vi "Request CORE.vi"(4 "Timeout":i32, 5 "Answer UE":refnum<user-event>, 6 "Response":bool, 7 "Write":refnum<queue>, 8 "Error In":errorcluster, 9 "Data":string, 10 "Function ID":u8, 11 "Stack ID":u8) -> (0 "Error Out":errorcluster, 1 "timed out":bool, 2 "Sucessful":bool, 3 "Answer":T1)   [LabVIEW 2011, in "Tinkerforge.lvlib" / "IP Connection.lvclass"]
doc: "This VI encapsulates the Request handling for the device class."
uses:
  IP Connection.lvclass
  Type Definitions/Message.ctl
  Type Definitions/Answer.ctl
  Type Definitions/Request Type.ctl
  Type Definitions/Errors.ctl
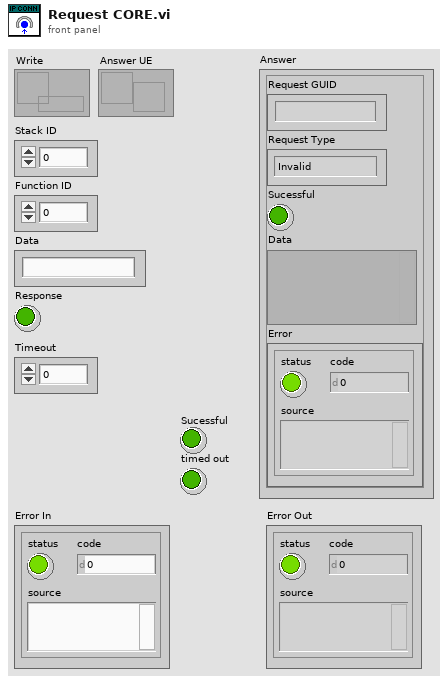
[diagram p1: front panel]
types:
  T1 = typedef "Tinkerforge.lvlib/IP Connection.lvclass/Answer.ctl" = cluster{"Request GUID":string, "Request Type":T2, "Sucessful":bool, "Data":variant, "Error":errorcluster}
  T2 = typedef "Tinkerforge.lvlib/IP Connection.lvclass/Request Type.ctl" = enum8{"Invalid", "Write"}
  T3 = typedef "Tinkerforge.lvlib/IP Connection.lvclass/Errors.ctl" = enum16{"Timeout", "Device type incorrect", "Device already added", "Device not existing"}
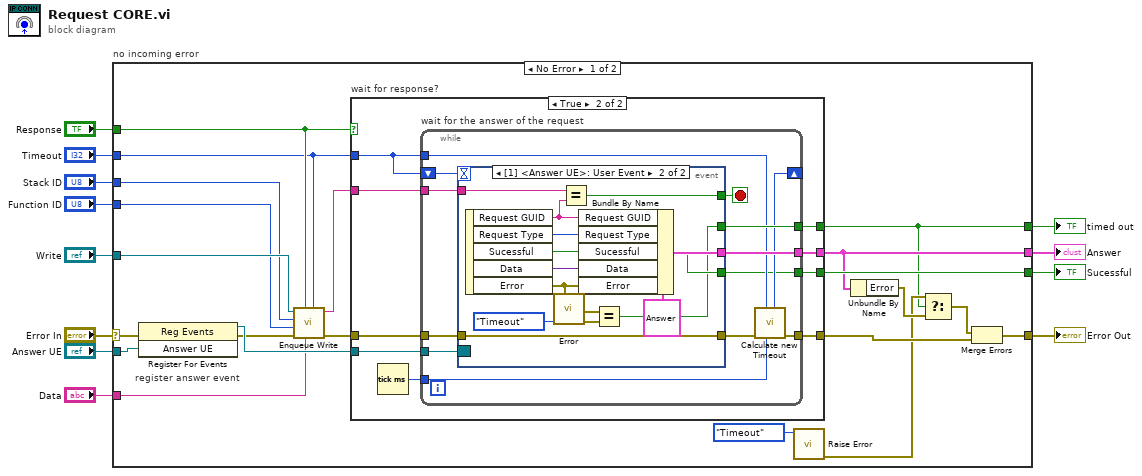
[diagram p0: block diagram]
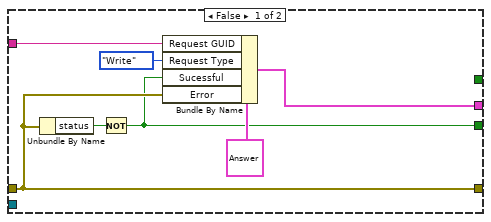
[diagram p2: hidden frame]
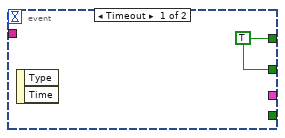
[diagram p3: hidden frame]
diagram:
  n1 = case "no incoming error" shown="No Error" "Error In" {
    selector: "Error In" -> [w29 w77]
    tunnel: [w19 w77] -> w11
    tunnel: "Write" -> [w28 _]
    tunnel: "Answer UE" -> [w33 _]
    tunnel: [w21 _] -> w8
    tunnel: [w14 _] -> w7
    tunnel: "Response" -> [w23 _]
    tunnel: "Stack ID" -> [w26 _]
    tunnel: "Data" -> [w25 _]
    tunnel: "Function ID" -> [w24 _]
    tunnel: "Timeout" -> [w18 _]
    tunnel: [w22 _] -> w1
    frame No Error {
      # "register answer event"
      n2 = register-events(error in=w29, w33) -> (reference out=w32:refnum<event-registration>, error out=w31:errorcluster)  [unwired: 1 in]
      n3 = call "Enqueue Write.vi"("Timeout"=w18, "Data"=w25, "Response"=w23, "error in (no error)"=w31, "Function ID"=w24, "Stack ID"=w26, "Write"=w28) -> ("error out"=w30:errorcluster, "GUID"=w27:string)  [unwired: 3 in]
      n4 = case "wait for response?" shown="True" w23 {
        tunnel: w32 -> [_ w49]
        tunnel: [w36 w48] -> w21
        tunnel: [_ w47] -> w14
        tunnel: [w38 w45] -> w20
        tunnel: w30 -> [w38 w44]
        tunnel: w27 -> [w40 w43]
        tunnel: w18 -> [_ w42]
        tunnel: [w34 w41] -> w22
        frame False {
          n5 = Unbundle By Name(w38) -> ("status"=w35:bool)
          n6 = Not(x=w35) -> (.not. x?=w34:bool)
          n7 = Bundle By Name(cluster=T1 {"Request GUID"="", "Request Type"=enum."Invalid", "Sucessful"=FALSE, "Data"=variant, "Error"={"status"=FALSE, "code"=0, "source"=""}} ("Answer"), "Request GUID"=w40, "Request Type"=Request_Type."Write", "Sucessful"=w34, "Error"=w38) -> (w36:T1)
        }
        frame True {
          n8 = Tick Count (ms)() -> (millisecond timer value=w46:u32)
          n9 = while "wait for the answer of the request" {
            tunnel: w44 -> [w60]
            tunnel: w49 -> [w62]
            shift-right: [w51] -> _
            shift-left: w42 -> [w61]
            tunnel: w43 -> [w59]
            tunnel: [w57] -> w48
            tunnel: [w56] -> w47
            tunnel: w46 -> [w53]
            tunnel: [w54] -> w45
            tunnel: w42 -> [w52]
            tunnel: [w50] -> w41
            stop <- w58 stop-if-true
            n10 = event shown="[1] <Answer UE>: User Event" {
              selector: w62 -> [_ _]
              dyn-events: _ -> [_ _]
              timeout: w61 -> [_ _]
              tunnel: w60 -> [_ w69]
              tunnel: w59 -> [_ w76]
              tunnel: [w63 w75] -> w58
              tunnel: [_ w70] -> w57
              tunnel: [w63 w64] -> w56
              tunnel: [_ w69] -> w55
              tunnel: [_ w68] -> w50
              event Timeout {
                w63 = TRUE
                n11 = event-data() -> ()  [unwired: 1 in, 2 out]
              }
              event User Event {
                n12 = event-data() -> ("Request GUID"=w73:string, "Request Type"=w72:T2, "Sucessful"=w68:bool, "Data"=w71:variant, "Error"=w67:errorcluster)  [unwired: 1 in]
                n13 = call "Error.vi"("Error"=Errors."Timeout") -> ("error cluster"=w65:errorcluster)  [unwired: 10 in]
                n14 = Equal?(x=w76, y=w73) -> (x = y?=w75:bool)
                n15 = Bundle By Name(cluster=T1 {"Request GUID"="", "Request Type"=enum."Invalid", "Sucessful"=FALSE, "Data"=variant, "Error"={"status"=FALSE, "code"=0, "source"=""}} ("Answer"), "Request GUID"=w73, "Request Type"=w72, "Sucessful"=w68, "Data"=w71, "Error"=w67) -> (w70:T1)
                n16 = Equal?(x=w67, y=w65) -> (x = y?=w64:bool)
              }
            }
            n17 = call "Calculate new Timeout.vi"("Start Time"=w53, "Total Timeout"=w52, "Error In"=w55) -> ("Error Out"=w54:errorcluster, "remaining Timeout"=w51:i32)  [unwired: 7 in]
          }
        }
      }
      n18 = call "Raise Error.vi"("Error"=Errors."Timeout") -> ("Error Out"=w15:errorcluster)  [unwired: 10 in]
      n19 = Unbundle By Name(w21) -> ("Error"=w17:errorcluster)
      n20 = Select(t=w15, s=w14, f=w17) -> (s? t:f=w13:errorcluster)
      n21 = Merge Errors(w13, w20) -> (w19:errorcluster)
    }
    frame Error {
    }
  }
  "Error Out" <- w11
  "timed out" <- w7
  "Answer" <- w8
  "Sucessful" <- w1
